vi "Acquisition & Generation test UI.vi"() -> ()   [LabVIEW 2014]
uses:
  <vilib>/rvi/interface/nirviMethod/nirviMethod.xnode
  <vilib>/rvi/errors/niLvFpgaMergeErrorWithErrorCode.vi
  <vilib>/FPGAPlugInAG/Dynamic/niLvFpga_Run_Dynamic.vi
  <vilib>/rvi/interface/nirviCloseFPGA/nirviCloseFPGA.xnode
  <vilib>/rvi/interface/nirviOpenFPGA/nirviOpenFPGA.xnode
  Acquisition & Generation test.vi
  <vilib>/FPGAPlugInAG/Dynamic/niLvFpga_ConfigureFifo_Dynamic.vi
  <vilib>/FPGAPlugInAG/Dynamic/niLvFpga_StartFifo_Dynamic.vi
  <vilib>/FPGAPlugInAG/Dynamic/niLvFpga_ReadFifo_Dynamic.vi
  <vilib>/FPGAPlugInAG/Dynamic/niLvFpga_Close_Dynamic.vi
panel:
  out "Elements Remaining":u32
  out "Waveform Graph (input data)":dbl[](graph)
  in  "stop":bool
  in  "Number of Elements to read":u32=512
  in  "Wave path":path
  # "Generation"
  # "Acquisition"
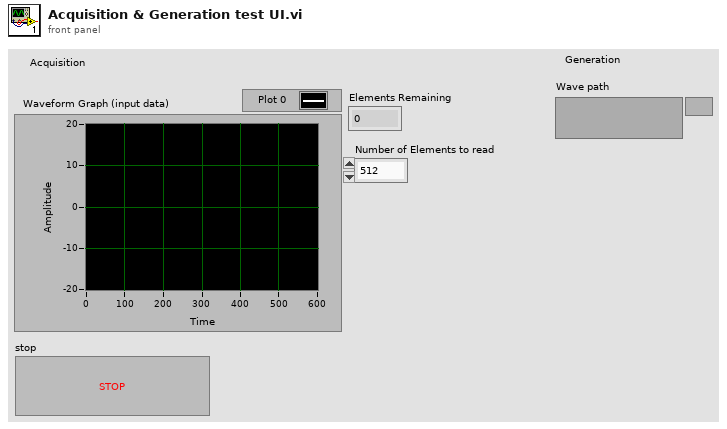
[diagram p1: front panel]
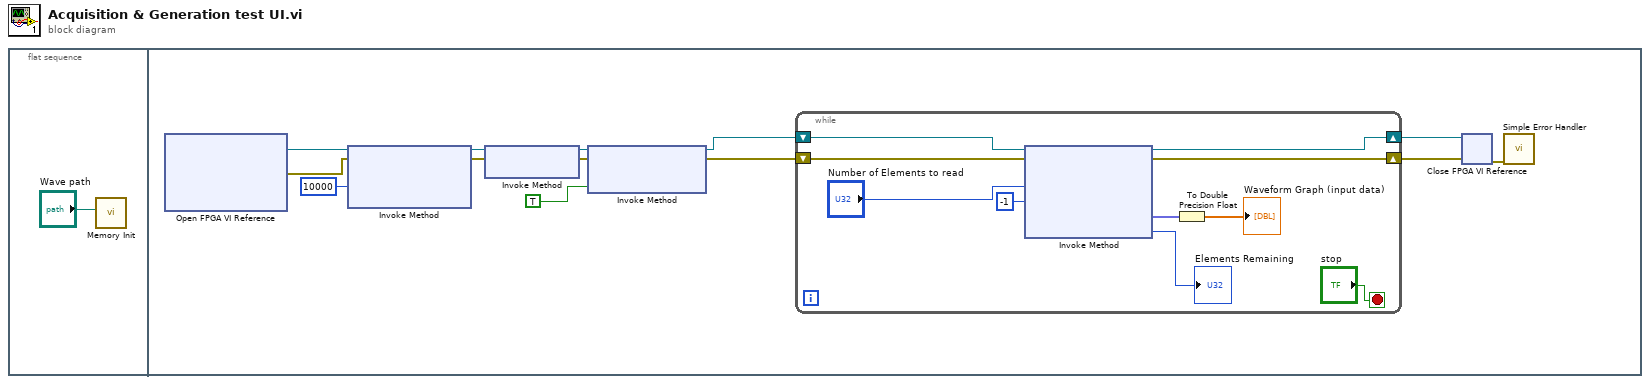
[diagram p0: block diagram]
diagram:
  n1 = flat-sequence {
    frame #0 {
      n2 = call "Memory Init.vi"("Wave path"="Wave path") -> ()  [unwired: 9 in]
    }
    frame #1 {
      n3 = xnode "Open FPGA VI Reference"() -> ("FPGA VI Reference Out"=w4:refnum<k20>, "error out"=w3:errorcluster)  [unwired: 2 in]
      n4 = xnode "Invoke Method"("FPGA VI Reference In"=w4, "error in"=w3, "Requested Depth"=u32 10000) -> ("FPGA VI Reference Out"=w14:refnum<k20>, "error out"=w13:errorcluster)  [unwired: 1 out]
      n5 = xnode "Invoke Method"("FPGA VI Reference In"=w14, "error in"=w13) -> ("FPGA VI Reference Out"=w11:refnum<k20>, "error out"=w10:errorcluster)
      n6 = xnode "Invoke Method"("FPGA VI Reference In"=w11, "error in"=w10, "Wait Until Done (F)"=TRUE) -> ("FPGA VI Reference Out"=w9:refnum<k20>, "error out"=w8:errorcluster)
      n7 = while {
        shift-right: [w16] -> w7
        shift-left: w9 -> [w22]
        shift-right: [w15] -> w6
        shift-left: w8 -> [w21]
        stop <- "stop" stop-if-true
        n8 = xnode "Invoke Method"("FPGA VI Reference In"=w22, "error in"=w21, "Number of Elements"="Number of Elements to read", "Timeout (ms)"=-1) -> ("FPGA VI Reference Out"=w16:refnum<k20>, "error out"=w15:errorcluster, "Data"=w19:fxp<+/-,12,5>[], "Elements Remaining"=→"Elements Remaining":u32)
        n9 = To Double Precision Float(number=w19) -> (double precision float=→"Waveform Graph (input data)":dbl[])
      }
      n10 = xnode "Close FPGA VI Reference"("FPGA VI Reference In"=w7, "error in"=w6) -> ("error out"=w5:errorcluster)
      n11 = call <vilib>:"Simple Error Handler.vi"("error in (no error)"=w5) -> ()  [unwired: 4 in, 5 out]
    }
  }
